vi "Tools_KeyedArray Clear.vi"(7 "array in":T1) -> (3 "array out":T1)   [LabVIEW 2012]
doc: "Returns an empty keyed array."
uses:
  Tools_KeyedArray KeyedArray.ctl
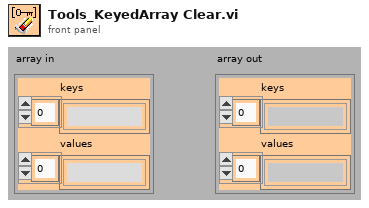
[diagram p1: front panel]
types:
  T1 = typedef "Tools_KeyedArray KeyedArray.ctl" = cluster{"keys":string[], "values":string[]}
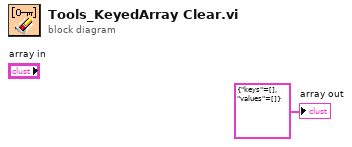
[diagram p0: block diagram]
diagram:
  "array out" <- cluster{"keys":string[], "values":string[]} {"keys"=[], "values"=[]} ("array out")
